vi "MDAQ_ReadAll.vi"(8 "error in":errorcluster, 11 "VISA resource name":refnum<visa-resource-name>) -> (0 "error IO":errorcluster, 1 "Buffer Not Empty":bool, 2 "read buffer":string, 3 "VISA resource name out":refnum<visa-resource-name>)   [LabVIEW 2021]
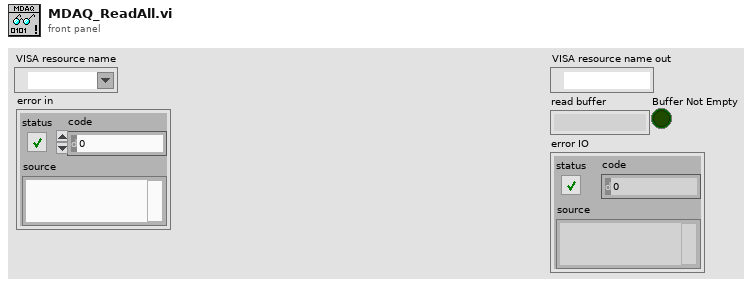
[diagram p1: front panel]
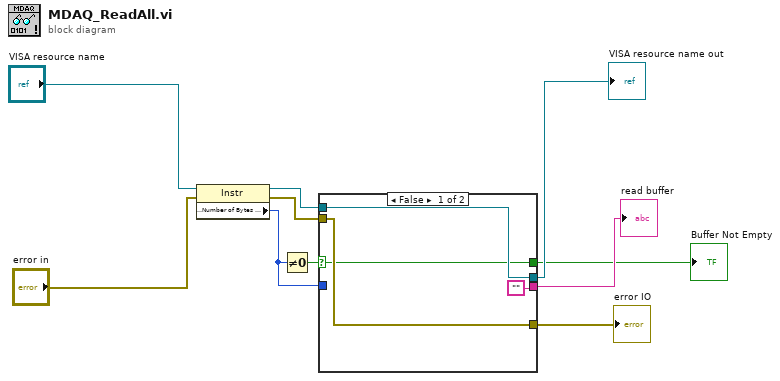
[diagram p0: block diagram]
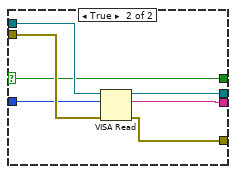
[diagram p2: hidden frame]
diagram:
  n1 = property class="Instr"(reference="VISA resource name", error in="error in") -> (reference out=w4:refnum<visa-resource-name>, error out=w7:errorcluster, "Serial Settings:Number of Bytes at Serial Port"=w6:u32)
  n2 = Not Equal To 0?(x=w6) -> (x != 0?=w8:bool)
  n3 = case shown="False" w8 {
    selector: w8 -> [w11 w15]
    tunnel: w7 -> [w12 w21]
    tunnel: w6 -> [_ w20]
    tunnel: [w13 w19] -> w3
    tunnel: ["" w18] -> w5
    tunnel: [w12 w17] -> w2
    tunnel: w4 -> [w13 w16]
    tunnel: [w11 w15] -> w1
    frame False {
    }
    frame True {
      n4 = VISA Read(VISA resource name=w16, byte count=w20, error in (no error)=w21) -> (VISA resource name out=w19:refnum<visa-resource-name>, read buffer=w18:string, error out=w17:errorcluster)  [unwired: 1 out]
    }
  }
  "VISA resource name out" <- w3
  "read buffer" <- w5
  "error IO" <- w2
  "Buffer Not Empty" <- w1
